vi "Translator.File.Order.vi"(8 "error in":errorcluster, 11 "Translation folder":path=path "D:/PL_0125_Sapphire_Automation_branches/SOFTWARE_v1.1-Translation/settings/Translation-Chinese.ini") -> (0 "error out":errorcluster)   [LabVIEW 2019, in "Tools.lvlib"]
uses:
  Tools.lvlib
  Tma.lib/nlconfig.llb/nlWrite Section (str).vi
  Tma.lib/nlconfig.llb/nlRead Section (str).vi
panel:
  out "section names":string[](array[string])
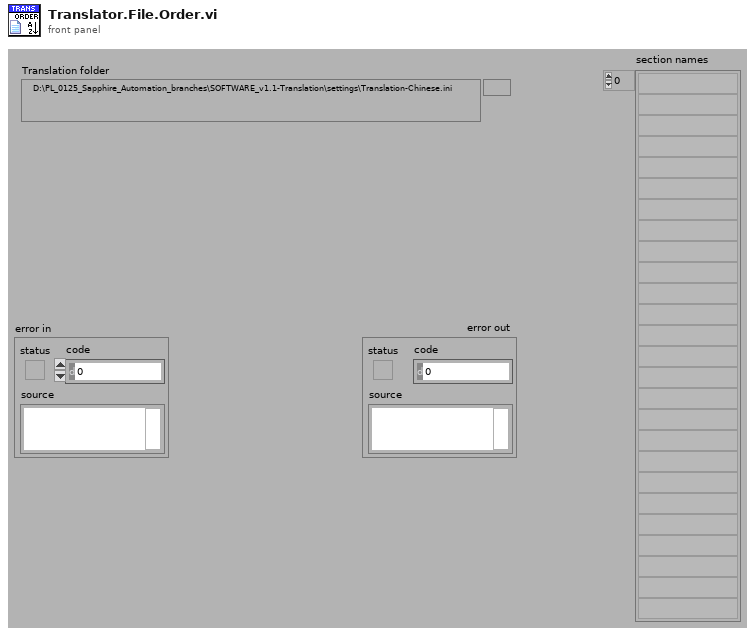
[diagram p1: front panel]
types:
  T1 = typedef "Tools.lvlib/nlConfig Data RefNum.ctl" = refnum<k4>
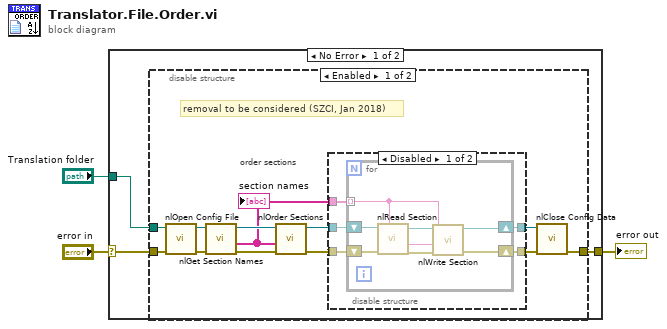
[diagram p0: block diagram]
diagram:
  n1 = case shown="No Error" "error in" {
    selector: "error in" -> [w5 w35]
    tunnel: "Translation folder" -> [w6 _]
    tunnel: [w4 w35] -> w2
    frame No Error {
      n2 = disable-structure shown="Enabled" {
        disable-tunnel: w6 -> [w14 _]
        disable-tunnel: w5 -> [w13 w34]
        disable-tunnel: [w12 w34] -> w4
        frame Enabled {
          # "removal to be considered (SZCI, Jan 2018)"
          # "order sections"
          n3 = call "nlOpen Config File.vi"("error in (no error)"=w13, "configuration file path"=w14) -> ("error out"=w15:errorcluster, "refnum"=w16:T1)  [unwired: 8 in]
          n4 = call "nlGet Section Names.vi"("error in (no error)"=w15, "refnum"=w16) -> ("error out"=w17:errorcluster, "section names"=w8:string[], "refnum out"=w18:T1)  [unwired: 7 in]
          "section names" <- w8
          n5 = call "nlOrder Sections.vi"("error in (no error)"=w17, "section names"=w8, "refnum"=w18) -> ("error out"=w11:errorcluster, "refnum out"=w10:T1)  [unwired: 7 in]
          n6 = disable-structure shown="Disabled" {
            disable-tunnel: w11 -> [w23 w32]
            disable-tunnel: w10 -> [w22 w33]
            disable-tunnel: [w21 w33] -> w9
            disable-tunnel: w8 -> [w20 _]
            disable-tunnel: [w19 w32] -> w7
            frame Disabled {
              n7 = for {
                tunnel: w20 -> [w26] mode=indexing
                shift-right: [w24] -> w21
                shift-left: w22 -> [w30]
                shift-right: [w25] -> w19
                shift-left: w23 -> [w31]
                n8 = call-poly "nlRead Section.vi"("sectionname"=w26, "error in (no error)"=w31, "refnum"=w30) -> ("error out"=w29:errorcluster, "contents out"=w28:string, "refnum out"=w27:T1)  [unwired: 5 in, 1 out]
                n9 = call-poly "nlWrite Section.vi"("sectionname"=w26, "error in (no error)"=w29, "contents in"=w28, "refnum"=w27) -> ("error out"=w25:errorcluster, "refnum out"=w24:T1)  [unwired: 5 in, 1 out]
              }
            }
            frame Enabled {
            }
          }
          n10 = call "nlClose Config Data.vi"("error in (no error)"=w7, "refnum"=w9) -> ("error out"=w12:errorcluster)  [unwired: 8 in, 1 out]
        }
        frame Disabled {
        }
      }
    }
    frame Error {
    }
  }
  "error out" <- w2
